vi "AO_AI_Task_4channels.vi"(6 "OSC Configuration":T3(array[cluster])=[{"Signal Type"=enum."Sine Wave", "DC"=0.0, "Amplitude"=0.1, "frequency"=20.0, "Phase"=0.0}, {"Signal Type"=enum."Sine Wave", "DC"=0.0, "Amplitude"=0.19999999999999993, "frequency"=20.0, "Phase"=0.0}, {"Signal Type"=enum."Sine Wave", "DC"=0.0, "Amplitude"=0.30000000000000004, "frequency"=20.0, "Phase"=0.0}, {"Signal Type"=enum."Sine Wave", "DC"=0.0, "Amplitude"=0.4, "frequency"=20.0, "Phase"=0.0}] {"frequency" format="%0.2p"; "Amplitude" format="%0.2p"; "DC" format="%.2p"}, 7 "AO Configuration":T1(array[cluster])=[{"Output physical channels"="PXI1Slot2/ao0:1", "AO. Max"=10.0, "AO.Min"=-10.0}, {"Output physical channels"="PXI1Slot3/ao0:1", "AO. Max"=10.0, "AO.Min"=-10.0}], 8 "AI Configuration":T2(array[cluster])=[{"AI Rate"=200000.0, "AI Block Size"=20000, "AI Buffer Size (s)"=10, "AI.Coupling"=10050, "AI.Max"=10.0, "AI.Min"=-10.0, "Input physical channels"="PXI1Slot2/ai0:1"}, {"AI Rate"=200000.0, "AI Block Size"=20000, "AI Buffer Size (s)"=10, "AI.Coupling"=10050, "AI.Max"=10.0, "AI.Min"=-10.0, "Input physical channels"="PXI1Slot3/ai0:1"}] {"AI.Coupling" items=["AC"=10045, "DC"=10050, "GND"=10066]; "AI Rate" format="%.2f"}) -> (0 "Sampling information":cluster{"Fs":dbl, "#s":dbl}[](array[cluster])=[{"Fs"=200000.00004074536, "#s"=20000.0}], 1 "Actual AI rate":dbl[](array[numeric])=[200000.00004074536], 2 "AO Task":refnum<k21>[](array[refnum]), 3 "AI task":refnum<k21>[](array[refnum]))   [LabVIEW 2011]
uses:
  <vilib>/DAQmx/write.llb/DAQmx Write (Analog 1D Wfm NChan NSamp).vi
  <vilib>/DAQmx/create/channels.llb/DAQmx Create Channel (AI-Voltage-Basic).vi
  <vilib>/DAQmx/configure/timing.llb/DAQmx Timing (Sample Clock).vi
  <vilib>/DAQmx/create/channels.llb/DAQmx Create Channel (AO-Voltage-Basic).vi
  <vilib>/DAQmx/configure/trigger.llb/DAQmx Start Trigger (Digital Edge).vi
  <vilib>/DAQmx/miscellaneous.llb/DAQmx Fill In Error Info.vi
  C:/Program Files (x86)/National Instruments/LabVIEW 2011/resource/objmgr/daqmx.rc
  <vilib>/measure/NI_MABase.lvlib
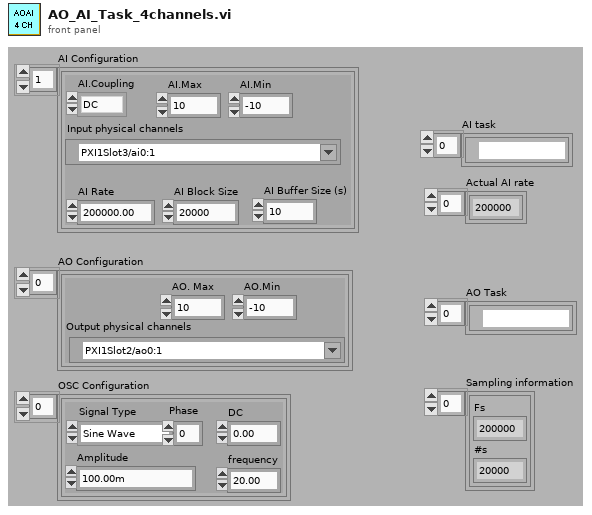
[diagram p1: front panel]
types:
  T1 = cluster{"Output physical channels":tag, "AO. Max":dbl, "AO.Min":dbl}[]
  T2 = cluster{"AI Rate":dbl, "AI Block Size":i32, "AI Buffer Size (s)":i32, "AI.Coupling":i32, "AI.Max":dbl, "AI.Min":dbl, "Input physical channels":tag}[]
  T3 = cluster{"Signal Type":enum16{"Sine Wave", "Triangle Wave", "Square Wave", "Sawtooth Wave"}, "DC":dbl, "Amplitude":dbl, "frequency":dbl, "Phase":dbl}[]
  T4 = cluster{"Signal Type":enum16{"Sine Wave", "Triangle Wave", "Square Wave", "Sawtooth Wave"}, "DC":dbl, "Amplitude":dbl, "frequency":dbl, "Phase":dbl}
  T5 = enum16{"Sine Wave", "Triangle Wave", "Square Wave", "Sawtooth Wave"}
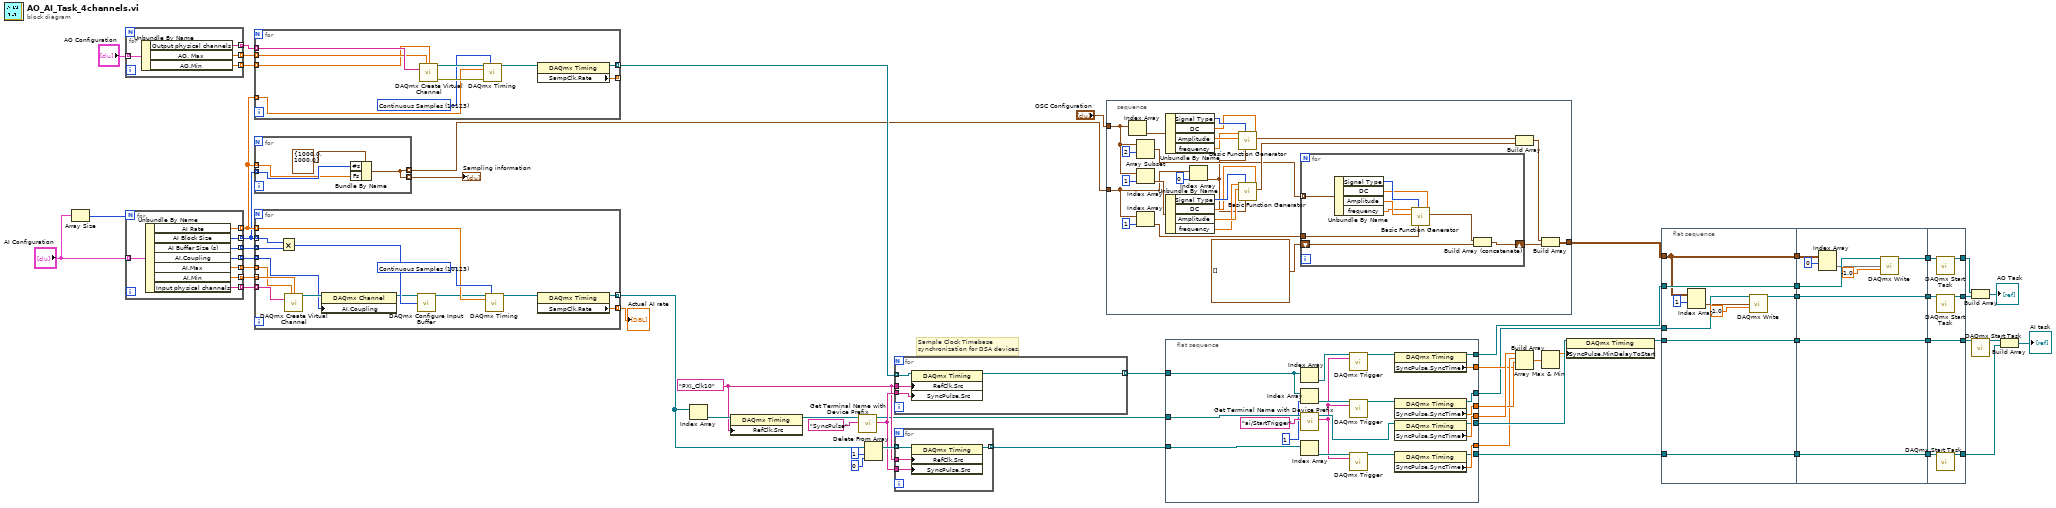
[diagram p0: block diagram]
diagram:
  w30 = tag "PXI_Clk10" ("RefClk.Src")
  # "Sample Clock Timebase \nsynchronization for DSA devices."
  n1 = Array Size(array="AI Configuration") -> (size(s)=w58:i32)
  n2 = for {
    tunnel: "AO Configuration" -> [w62] mode=indexing
    tunnel: [w61] -> w53 mode=indexing
    tunnel: [w60] -> w52 mode=indexing
    tunnel: [w59] -> w51 mode=indexing
    n3 = Unbundle By Name(w62) -> ("Output physical channels"=w61:tag, "AO. Max"=w60:dbl, "AO.Min"=w59:dbl)
  }
  n4 = for {
    N: w58 -> [_]
    tunnel: "AI Configuration" -> [w70] mode=indexing
    tunnel: [w69] -> w48 mode=indexing
    tunnel: [w68] -> w56 mode=indexing
    tunnel: [w67] -> w55 mode=indexing
    tunnel: [w66] -> w28 mode=indexing
    tunnel: [w65] -> w27 mode=indexing
    tunnel: [w64] -> w50 mode=indexing
    tunnel: [w63] -> w34 mode=indexing
    n5 = Unbundle By Name(w70) -> ("AI Rate"=w66:dbl, "AI Block Size"=w65:i32, "AI Buffer Size (s)"=w64:i32, "AI.Coupling"=w63:i32, "AI.Max"=w67:dbl, "AI.Min"=w68:dbl, "Input physical channels"=w69:tag)
  }
  n6 = for {
    tunnel: w53 -> [w80] mode=indexing
    tunnel: w52 -> [w79] mode=indexing
    tunnel: w51 -> [w78] mode=indexing
    tunnel: [w74] -> w42 mode=indexing
    tunnel: [w73] -> _ mode=indexing
    tunnel: w28 -> [w71] mode=indexing
    w72 = 10123 items=["Finite Samples"=10178, "Continuous Samples"=10123, "Hardware Timed Single Point"=12522] ("sample mode")
    n7 = call-poly <vilib>:"DAQmx Create Virtual Channel.vi"("maximum value"=w79, "minimum value"=w78, "physical channels"=w80) -> ("task out"=w77:refnum<k21>, "error out"=w76:errorcluster)  [unwired: 11 in]
    n8 = call-poly <vilib>:"DAQmx Timing.vi"("task/channels in"=w77, "sample mode"=w72, "rate"=w71, "error in"=w76) -> ("task out"=w75:refnum<k21>)  [unwired: 10 in, 1 out]
    n9 = property class="DAQmx Timing"(reference=w75) -> (reference out=w74:refnum<k21>, "SampClk.Rate"=w73:dbl)  [unwired: 1 in, 1 out]
  }
  n10 = for {
    tunnel: w28 -> [w83] mode=indexing
    tunnel: w27 -> [w84] mode=indexing
    tunnel: [w81] -> w26 mode=indexing
    tunnel: [w81] -> w25 mode=indexing
    n11 = Bundle By Name(cluster=cluster{"Fs":dbl, "#s":dbl} {"Fs"=1000.0, "#s"=1000.0} ("sampling info"), "#s"=w84, "Fs"=w83) -> (w81:cluster{"Fs":dbl, "#s":dbl})
  }
  "Sampling information" <- w26
  n12 = for {
    tunnel: w48 -> [w99] mode=indexing
    tunnel: w56 -> [w98] mode=indexing
    tunnel: w55 -> [w97] mode=indexing
    tunnel: w28 -> [w95] mode=indexing
    tunnel: w27 -> [w93] mode=indexing
    tunnel: w50 -> [w92] mode=indexing
    tunnel: [w89] -> w49 mode=indexing
    tunnel: [w88] -> w47 mode=indexing
    tunnel: w34 -> [w85] mode=indexing
    w96 = 10123 items=["Finite Samples"=10178, "Continuous Samples"=10123, "Hardware Timed Single Point"=12522] ("sample mode")
    n13 = Multiply(x=w93, y=w92) -> (x*y=w91:i32)
    n14 = call-poly <vilib>:"DAQmx Create Virtual Channel.vi"("maximum value"=w97, "minimum value"=w98, "physical channels"=w99) -> ("task out"=w87:refnum<k21>)  [unwired: 11 in, 1 out]
    n15 = property class="DAQmx Channel"(reference=w87, "AI.Coupling"=w85) -> (reference out=w86:refnum<k21>)  [unwired: 1 in, 1 out]
    n16 = call <vilib>:"DAQmx Configure Input Buffer.vi"("task/channels in"=w86, "buffer size (in samples per channel)"=w91) -> ("task out"=w94:refnum<k21>)  [unwired: 12 in, 1 out]
    n17 = call-poly <vilib>:"DAQmx Timing.vi"("task/channels in"=w94, "sample mode"=w96, "rate"=w95) -> ("task out"=w90:refnum<k21>)  [unwired: 11 in, 1 out]
    n18 = property class="DAQmx Timing"(reference=w90) -> (reference out=w88:refnum<k21>, "SampClk.Rate"=w89:dbl)  [unwired: 1 in, 1 out]
  }
  "Actual AI rate" <- w49
  n19 = Index Array(array=w47) -> (element=w32:refnum<k21>)  [unwired: 1 in]
  n20 = property class="DAQmx Timing"(reference=w32, "RefClk.Src"=w30) -> (reference out=w31:refnum<k21>)  [unwired: 1 in, 1 out]
  n21 = call "Get Terminal Name with Device Prefix.vi"("Local Terminal Name"="SyncPulse", "task/channels in"=w31) -> ("Terminal Name with Device Prefix"=w41:tag, "task out"=w24:refnum<k21>)  [unwired: 7 in, 1 out]
  n22 = Delete From Array(array=w47, length=1, index=0) -> (array with subset deleted=w43:refnum<k21>[])  [unwired: 1 out]
  n23 = for {
    tunnel: w42 -> [w103] mode=indexing
    tunnel: w30 -> [w102]
    tunnel: w41 -> [w101]
    tunnel: [w100] -> w39 mode=indexing
    n24 = property class="DAQmx Timing"(reference=w103, "RefClk.Src"=w102, "SyncPulse.Src"=w101) -> (reference out=w100:refnum<k21>)  [unwired: 1 in, 1 out]
  }
  n25 = for {
    tunnel: w43 -> [w107] mode=indexing
    tunnel: w30 -> [w106]
    tunnel: w41 -> [w105]
    tunnel: [w104] -> w40 mode=indexing
    n26 = property class="DAQmx Timing"(reference=w107, "RefClk.Src"=w106, "SyncPulse.Src"=w105) -> (reference out=w104:refnum<k21>)  [unwired: 1 in, 1 out]
  }
  n27 = stacked-sequence {
    tunnel: "OSC Configuration" -> [w119]
    tunnel: [w116] -> w9
    tunnel: w25 -> [w109]
    frame #0 {
      n28 = Index Array(array=w119) -> (element=w131:T4)  [unwired: 1 in]
      n29 = Array Subset(array=w119, index=2) -> (w117:T3)  [unwired: 1 in]
      n30 = Index Array(array=w119, index=1) -> (element=w130:T4)
      n31 = Index Array(array=w109, index=1) -> (element=w108:cluster{"Fs":dbl, "#s":dbl})
      n32 = Unbundle By Name(w131) -> ("Signal Type"=w129:T5, "DC"=w128:dbl, "Amplitude"=w127:dbl, "frequency"=w126:dbl)
      n33 = Unbundle By Name(w130) -> ("Signal Type"=w125:T5, "DC"=w124:dbl, "Amplitude"=w123:dbl, "frequency"=w122:dbl)
      n34 = Index Array(array=w109, index=0) -> (element=w110:cluster{"Fs":dbl, "#s":dbl})
      n35 = call <vilib>:"Basic Function Generator.vi"("offset"=w128, "sampling info"=w110, "signal type"=w129, "amplitude"=w127, "frequency"=w126) -> ("signal out"=w121:waveform(dbl))  [unwired: 4 in, 2 out]
      n36 = call <vilib>:"Basic Function Generator.vi"("offset"=w124, "sampling info"=w110, "signal type"=w125, "amplitude"=w123, "frequency"=w122) -> ("signal out"=w120:waveform(dbl))  [unwired: 4 in, 2 out]
      n37 = for {
        tunnel: w117 -> [w141] mode=indexing
        shift-right: [w136] -> w114
        shift-left: waveform(dbl)[] [] -> [w135]
        tunnel: w108 -> [w133]
        n38 = Unbundle By Name(w141) -> ("Signal Type"=w140:T5, "DC"=w139:dbl, "Amplitude"=w138:dbl, "frequency"=w137:dbl)
        n39 = call <vilib>:"Basic Function Generator.vi"("offset"=w139, "sampling info"=w133, "signal type"=w140, "amplitude"=w138, "frequency"=w137) -> ("signal out"=w134:waveform(dbl))  [unwired: 4 in, 2 out]
        n40 = Build Array (concatenate)(w134, w135) -> (w136:waveform(dbl)[])
      }
      n41 = Build Array(w121, w120) -> (w113:waveform(dbl)[])
      n42 = Build Array(w113, w114) -> (w116:waveform(dbl)[][])
    }
  }
  n43 = flat-sequence {
    tunnel: w40 -> [w154]
    tunnel: w39 -> [w148]
    tunnel: [w162] -> w38
    tunnel: [w161] -> w36
    tunnel: [w160] -> w33
    tunnel: [w159] -> w10
    tunnel: w24 -> [w155]
    tunnel: [w145] -> w23
    tunnel: [w144] -> w22
    tunnel: [w143] -> w12
    tunnel: [w142] -> w11
    frame #0 {
      n44 = Index Array(array=w148) -> (element=w152:refnum<k21>)  [unwired: 1 in]
      n45 = Index Array(array=w148, index=1) -> (element=w147:refnum<k21>)
      n46 = call "Get Terminal Name with Device Prefix.vi"("Local Terminal Name"="ai/StartTrigger", "task/channels in"=w155) -> ("Terminal Name with Device Prefix"=w146:tag, "task out"=w157:refnum<k21>)  [unwired: 7 in, 1 out]
      n47 = Index Array(array=w154) -> (element=w153:refnum<k21>)  [unwired: 1 in]
      n48 = call-poly <vilib>:"DAQmx Trigger.vi"("task/channels in"=w152, "source"=w146) -> ("task out"=w150:refnum<k21>)  [unwired: 12 in, 1 out]
      n49 = call-poly <vilib>:"DAQmx Trigger.vi"("task/channels in"=w147, "source"=w146) -> ("task out"=w158:refnum<k21>)  [unwired: 12 in, 1 out]
      n50 = call-poly <vilib>:"DAQmx Trigger.vi"("task/channels in"=w153, "source"=w146) -> ("task out"=w151:refnum<k21>)  [unwired: 12 in, 1 out]
      n51 = property class="DAQmx Timing"(reference=w150) -> (reference out=w142:refnum<k21>, "SyncPulse.SyncTime"=w144:dbl)  [unwired: 1 in, 1 out]
      n52 = property class="DAQmx Timing"(reference=w158) -> (reference out=w159:refnum<k21>, "SyncPulse.SyncTime"=w160:dbl)  [unwired: 1 in, 1 out]
      n53 = property class="DAQmx Timing"(reference=w157) -> (reference out=w161:refnum<k21>, "SyncPulse.SyncTime"=w162:dbl)  [unwired: 1 in, 1 out]
      n54 = property class="DAQmx Timing"(reference=w151) -> (reference out=w143:refnum<k21>, "SyncPulse.SyncTime"=w145:dbl)  [unwired: 1 in, 1 out]
    }
  }
  n55 = Build Array(w38, w23, w33, w22) -> (w37:dbl[])
  n56 = Array Max & Min(array=w37) -> (max value=w35:dbl)  [unwired: 3 out]
  n57 = property class="DAQmx Timing"(reference=w36, "SyncPulse.MinDelayToStart"=w35) -> (reference out=w13:refnum<k21>)  [unwired: 1 in, 1 out]
  n58 = flat-sequence {
    tunnel: w13 -> [w170]
    tunnel: w12 -> [w171]
    tunnel: [w171] -> w21
    tunnel: [w170] -> w20
    tunnel: [w169] -> w19
    tunnel: w11 -> [w169]
    tunnel: w10 -> [w168]
    tunnel: [w167] -> w18
    tunnel: w9 -> [w164]
    tunnel: [w164] -> w8
    tunnel: [w180] -> w17
    tunnel: [w179] -> w16
    tunnel: w21 -> [w180]
    tunnel: w20 -> [w179]
    tunnel: w19 -> [w178]
    tunnel: [w177] -> w15
    tunnel: w18 -> [w177]
    tunnel: [w176] -> w14
    tunnel: w8 -> [w175]
    tunnel: [w184] -> w3
    tunnel: [w185] -> w2
    tunnel: [w186] -> w5
    tunnel: [w183] -> w7
    tunnel: w17 -> [w187]
    tunnel: w16 -> [w183]
    tunnel: w15 -> [w182]
    tunnel: w14 -> [w181]
    frame #0 {
      n59 = Index Array(array=w164, index (row)=1) -> (element=w165:waveform(dbl)[])  [unwired: 1 in]
      n60 = call-poly <vilib>:"DAQmx Write.vi"("task/channels in"=w168, "data"=w165, "timeout"=-1.0) -> ("task out"=w167:refnum<k21>)  [unwired: 10 in, 2 out]
    }
    frame #1 {
      n61 = Index Array(array=w175, index (row)=0) -> (element=w173:waveform(dbl)[])  [unwired: 1 in]
      n62 = call-poly <vilib>:"DAQmx Write.vi"("task/channels in"=w178, "data"=w173, "timeout"=-1.0) -> ("task out"=w176:refnum<k21>)  [unwired: 10 in, 2 out]
    }
    frame #2 {
      n63 = call <vilib>:"DAQmx Start Task.vi"("task/channels in"=w181) -> ("task out"=w184:refnum<k21>)  [unwired: 13 in, 1 out]
      n64 = call <vilib>:"DAQmx Start Task.vi"("task/channels in"=w182) -> ("task out"=w185:refnum<k21>)  [unwired: 13 in, 1 out]
      n65 = call <vilib>:"DAQmx Start Task.vi"("task/channels in"=w187) -> ("task out"=w186:refnum<k21>)  [unwired: 13 in, 1 out]
    }
  }
  n66 = Build Array(w3, w2) -> (→"AO Task":refnum<k21>[])
  n67 = call <vilib>:"DAQmx Start Task.vi"("task/channels in"=w7) -> ("task out"=w6:refnum<k21>)  [unwired: 13 in, 1 out]
  n68 = Build Array(w6, w5) -> (→"AI task":refnum<k21>[])
